vi "DatasocketsPart2.vi"() -> ()   [LabVIEW 2016]
uses:
  <vilib>/Utility/file.llb/Read Delimited Spreadsheet (DBL).vi
  <vilib>/Platform/browser.llb/Open URL in Default Browser (string).vi
  <vilib>/gmath/NI_Gmath.lvlib
panel:
  in  "?":bool
  in  "?":bool
  out "See File":path
  out "Values":dbl[](array[numeric])
  out "Series Check":dbl
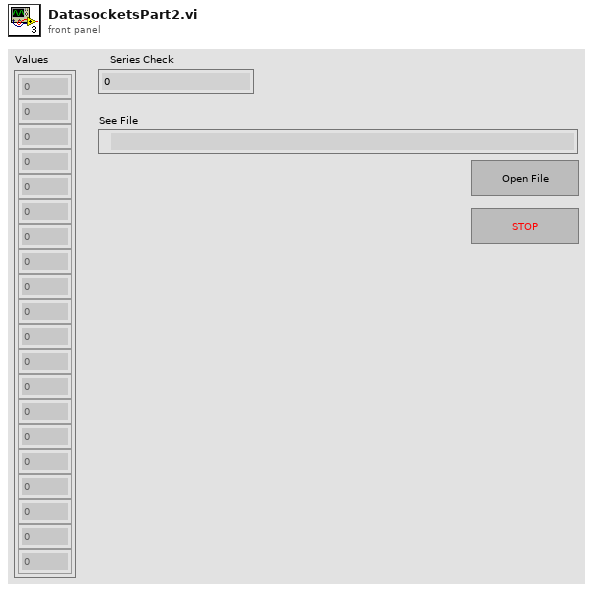
[diagram p1: front panel]
types:
  T1 = enum16{"open", "replace", "create", "open or create", "replace or create", "replace or create with confirmation"}
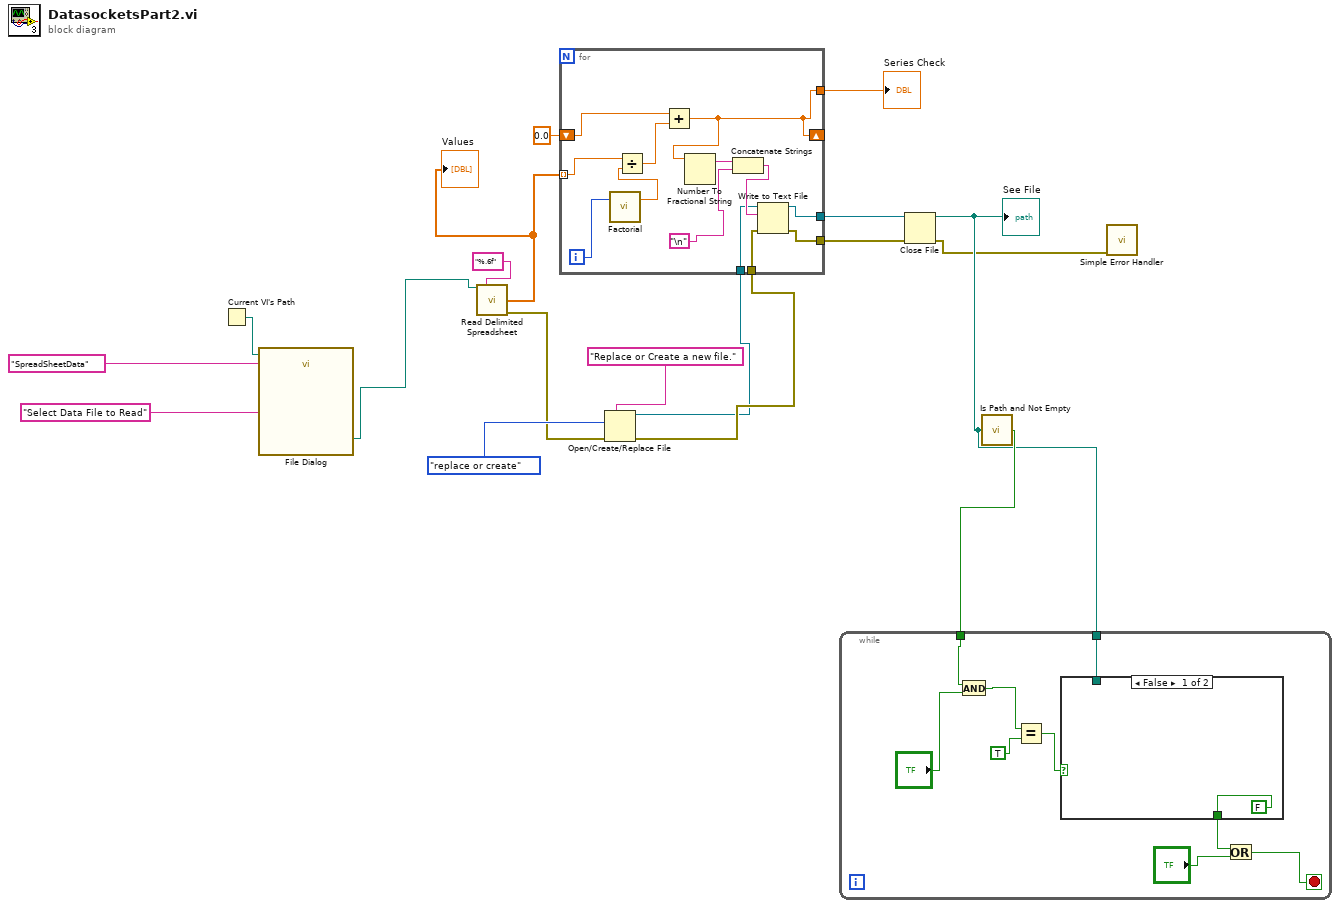
[diagram p0: block diagram]
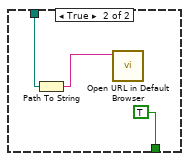
[diagram p2: hidden frame]
diagram:
  n1 = Current VI's Path() -> (path=w5:path)
  n2 = call "File Dialog"("start path"=w5, "prompt"="Select Data File to Read", "default name"="SpreadSheetData") -> ("selected path"=w1:path)  [unwired: 9 in, 3 out]
  n3 = call-poly <vilib>:"Read Delimited Spreadsheet.vi"("file path (dialog if empty)"=w1, "format (%.3f)"="%.6f" ("format string")) -> ("first row"=w9:dbl[], "error out"=w14:errorcluster)  [unwired: 8 in, 4 out]
  "Values" <- w9
  n4 = Open/Create/Replace File(error in=w14, prompt="Replace or Create a new file.", operation (0:open)=T1."replace or create") -> (refnum out=w2:refnum<file>, error out=w12:errorcluster)  [unwired: 3 in, 1 out]
  n5 = for {
    tunnel: w9 -> [w31] mode=indexing
    tunnel: w12 -> [w28]
    tunnel: [w25] -> w11
    shift-right: [w22] -> _
    shift-left: 0.0 -> [w24]
    tunnel: [w22] -> w7
    tunnel: [w20] -> w3
    tunnel: w2 -> [w19]
    i -> [w30]
    n6 = call <vilib>:"Factorial.vi"("n"=w30) -> ("n!"=w29:dbl)  [unwired: 2 in]
    n7 = Divide(x=w31, y=w29) -> (x/y=w23:dbl)
    n8 = Add(x=w24, y=w23) -> (x+y=w22:dbl)
    n9 = Number To Fractional String(number=w22) -> (F-format string=w27:string)  [unwired: 3 in]
    n10 = Concatenate Strings(w27, "\n") -> (w26:string)
    n11 = Write to Text File(file (use dialog)=w19, text=w26, error in=w28) -> (refnum out=w20:refnum<file>, error out=w25:errorcluster)  [unwired: 1 in, 1 out]
  }
  "Series Check" <- w7
  n12 = Close File(refnum=w3, error in=w11) -> (path=w17:path, error out=w10:errorcluster)
  "See File" <- w17
  n13 = call <vilib>:"Is Path and Not Empty.vi"("path"=w17) -> ("Is Path and Not Empty?"=w18:bool)  [unwired: 4 in]
  n14 = while {
    tunnel: w18 -> [w36]
    tunnel: w17 -> [w35]
    stop <- w32 stop-if-true
    n15 = And(x=w36, y="?") -> (x .and. y?=w39:bool)
    n16 = Equal?(x=w39, y=TRUE) -> (x = y?=w37:bool)
    n17 = case shown="False" w37 {
      tunnel: w35 -> [_ w43]
      tunnel: [FALSE TRUE] -> w33
      frame False {
      }
      frame True {
        n18 = Path To String(path=w43) -> (string=w44:string)
        n19 = call-poly <vilib>:"Open URL in Default Browser.vi"("URL"=w44) -> ()  [unwired: 5 in, 2 out]
      }
    }
    n20 = Or(x=w33, y="?") -> (x .or. y?=w32:bool)
  }
  n21 = call <vilib>:"Simple Error Handler.vi"("error in (no error)"=w10) -> ()  [unwired: 4 in, 5 out]
